vi "SetIOPulBase.vi"(8 "错误输入（无错误）":errorcluster, 9 "SelPinType":i32, 10 "nBase":u16) -> (0 "错误输出":errorcluster)   [LabVIEW 2014]
uses:
  X86Dll/ZXUTConfigMgr.dll
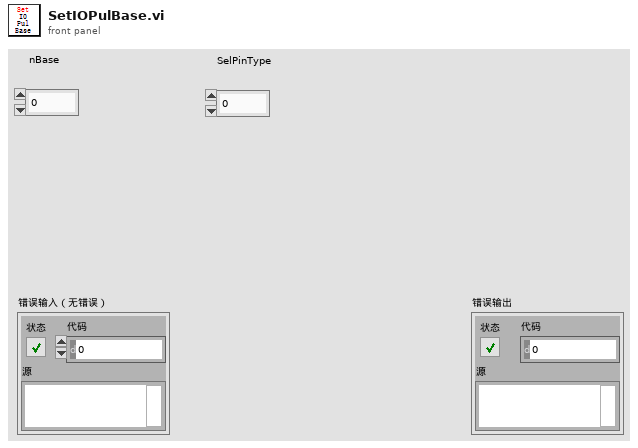
[diagram p1: front panel]
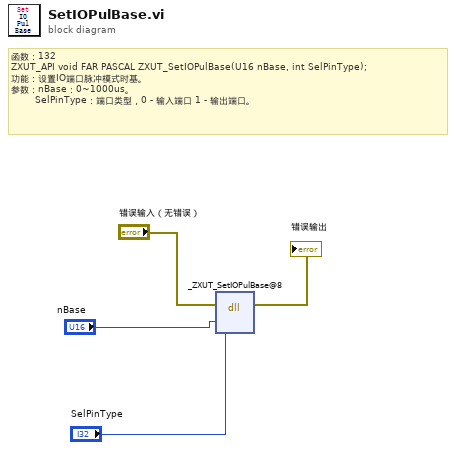
[diagram p0: block diagram]
diagram:
  # "函数：132\nZXUT_API void\tFAR PASCAL ZXUT_SetIOPulBase(U16 nBase, int SelPinType);\n功能：设置IO端口脉冲模式时基。\n参数：nBase：0~1000us。\n        SelPinType：端口类型，0 - 输入端口 1 - 输出端口。"
  n1 = dll-call lib="D:/Software/Utrasonic on-line monitoring/X86Dll/ZXUTConfigMgr.dll" fn="_ZXUT_SetIOPulBase@8"(error in="错误输入（无错误）", "nBase"="nBase", "SelPinType"="SelPinType") -> (error out=→"错误输出":errorcluster)  [unwired: 5 in, 1 out]
